vi "油动机名称.vi"() -> ()   [LabVIEW 2013]
panel:
  in  "油动机名称":string
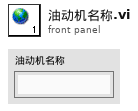
[diagram p1: front panel]
diagram:
